vi "FieldOrientedStateController.vi"(1 "Drive Mode":T1(ring)) -> (0 "Field Oriented":bool)   [LabVIEW 2019]
uses:
  <vilib>/Rock Robotics/WPI/DriverStation/WPI_DriverStationRobotMode2.ctl
  dsinstructions.vi
  dsdata.vi
  sensors.vi
  outputs.vi
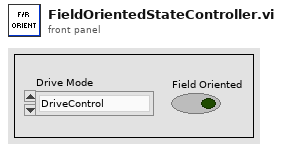
[diagram p1: front panel]
types:
  T1 = enum16{"DriveControl", "TargetControlH", "FeederStation"}
  T2 = typedef "WPI_DriverStationRobotMode2.ctl" = enum16{"Autonomous Disabled", "Autonomous Enabled", "Teleop Disabled", "Teleop Enabled", "Disconnected", "Finish", "Test Disabled", "Test Enabled", "Emergency Stopped"}
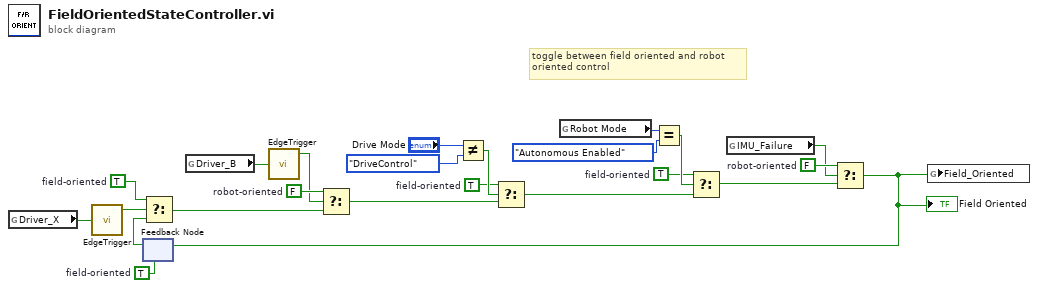
[diagram p0: block diagram]
diagram:
  w2 = TRUE  # field-oriented
  w9 = FALSE  # robot-oriented
  w20 = TRUE  # field-oriented
  w16 = TRUE  # field-oriented
  w15 = FALSE  # robot-oriented
  w14 = TRUE  # field-oriented
  # "toggle between field oriented and robot \noriented control"
  n1 = global read "dsinstructions.vi" "Driver_X"() -> (w13:bool)
  n2 = call "EdgeTrigger.vi"("Input Signal"=w13) -> ("Rising Edge Trigger"=w19:bool)  [unwired: 2 out]
  n3 = feedback #1(w14) -> (w18:bool)
  n4 = Select(t=w16, s=w19, f=w18) -> (s? t:f=w17:bool)
  n5 = global read "dsinstructions.vi" "Driver_B"() -> (w12:bool)
  n6 = call "EdgeTrigger.vi"("Input Signal"=w12) -> ("Rising Edge Trigger"=w7:bool)  [unwired: 2 out]
  n7 = Select(t=w15, s=w7, f=w17) -> (s? t:f=w4:bool)
  n8 = Not Equal?(x="Drive Mode", y=T1."DriveControl") -> (x != y?=w3:bool)
  n9 = Select(t=w2, s=w3, f=w4) -> (s? t:f=w1:bool)
  n10 = global read "dsdata.vi" "Robot Mode"() -> (w21:T2)
  n11 = Equal?(x=w21, y=WPI_DriverStationRobotMode2."Autonomous Enabled") -> (x = y?=w23:bool)
  n12 = Select(t=w20, s=w23, f=w1) -> (s? t:f=w11:bool)
  n13 = global read "sensors.vi" "IMU_Failure"() -> (w8:bool)
  n14 = Select(t=w9, s=w8, f=w11) -> (s? t:f=w10:bool)
  "Field Oriented" <- w10
  n15 = feedback-in #1(w10) -> ()
  n16 = global write "outputs.vi" "Field_Oriented"(w10) -> ()
